vi "SignalGenerator.vi"() -> ()   [LabVIEW 2015]
panel:
  out "error out":errorcluster
  in  "error in (no error)":errorcluster
  in  "Stop":bool
  in  "amplitude":dbl
  in  "frequency":dbl
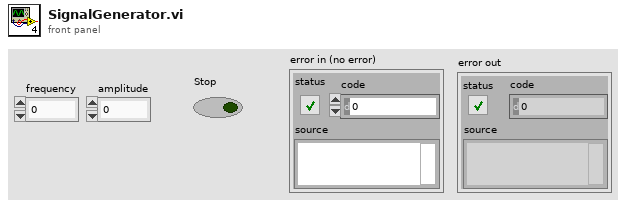
[diagram p1: front panel]
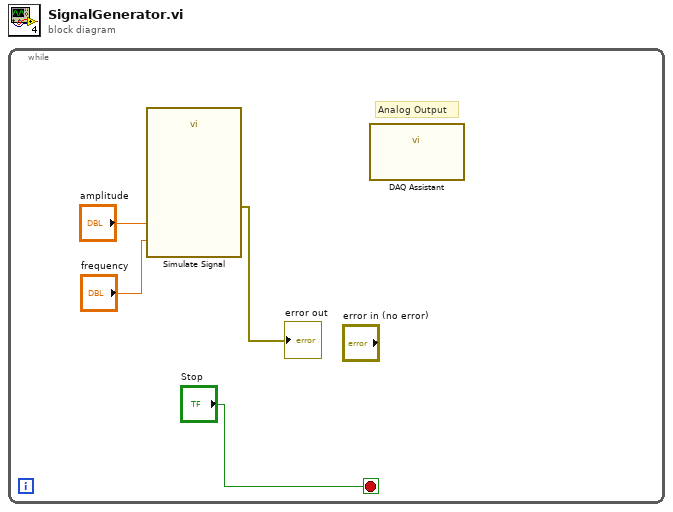
[diagram p0: block diagram]
diagram:
  n1 = while {
    stop <- "Stop" stop-if-true
    # "Analog Output"
    n2 = call "Simulate Signal"("Frequency"="frequency", "Amplitude"="amplitude") -> ("error out"=→"error out":errorcluster)  [unwired: 12 in, 1 out]
    n3 = call "DAQ Assistant"() -> ()  [unwired: 12 in]
  }
